vi "Check Connection.vi"(8 "error in (no error)":errorcluster, 11 "Connection In":refnum<k5>) -> (0 "error out":errorcluster, 1 "Disconnected":bool, 3 "Connection out":refnum<k5>)   [LabVIEW 2015]
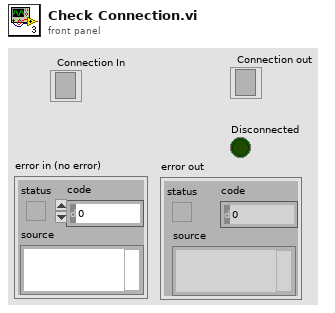
[diagram p1: front panel]
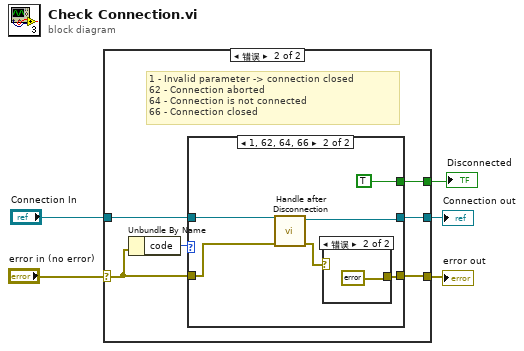
[diagram p0: block diagram]
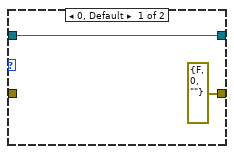
[diagram p3: hidden frame]
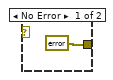
[diagram p4: hidden frame]
diagram:
  n1 = case shown="错误" "error in (no error)" {
    selector: "error in (no error)" -> [w7 w12]
    tunnel: [w7 w11] -> w4
    tunnel: "Connection In" -> [w6 w10]
    tunnel: [w6 w9] -> w2
    tunnel: [_ w8] -> w1
    frame No Error {
    }
    frame Error {
      # "1 - Invalid parameter -> connection closed\n62 - Connection aborted\n64 - Connection is not connected\n66 - Connection closed"
      n2 = Unbundle By Name(w12) -> ("code"=w13:i32)
      n3 = case shown="1, 62, 64, 66" w13 {
        tunnel: w12 -> [_ w18]
        tunnel: [errorcluster {"status"=FALSE, "code"=0, "source"=""} ("error IO") w17] -> w11
        tunnel: w10 -> [w15 w20]
        tunnel: [w15 w19] -> w9
        tunnel: [_ TRUE] -> w8
        frame 0, Default {
        }
        frame 1, 62, 64, 66 {
          n4 = call "Handle after Disconnection.vi"("error in (no error)"=w18, "Connection In"=w20) -> ("error out"=w16:errorcluster, "Connection out"=w19:refnum<k5>)  [unwired: 8 in]
          n5 = case shown="错误" w16 {
            tunnel: [errorcluster {"status"=FALSE, "code"=0, "source"=""} ("error IO") errorcluster {"status"=FALSE, "code"=0, "source"=""} ("error IO")] -> w17
            frame No Error {
            }
            frame Error {
            }
          }
        }
      }
    }
  }
  "error out" <- w4
  "Connection out" <- w2
  "Disconnected" <- w1
